vi "GrabNsvReadings.vi"(11 "Simulated Telemetry in":T1 {"Brake Pressure (PSI)" scale=0.0..1000.0; "Maglock 4 (mm)" scale=0.0..15.0; "Maglock 3 (mm)" scale=0.0..15.0; "Maglock 2 (mm)" scale=0.0..15.0; "Maglock 1 (mm)" scale=0.0..15.0; "ToF 4 (mm)" scale=0.0..100.0; "ToF 3 (mm)" scale=0.0..100.0; "ToF 2 (mm)" scale=0.0..100.0; "ToF 1 (mm)" scale=0.0..100.0; "Levitation Pressure (PSI)" scale=0.0..1000.0; "Utility Pressure (PSI)" scale=0.0..1000.0; "Tank Pressure (PSI)" scale=0.0..1000.0; "Brake Voltage (V)" scale=0.0..15.0; "Battery Voltage (V)" scale=0.0..15.0; "Brake Current (A)" scale=0.0..500.0; "Battery Current (A)" scale=0.0..500.0}) -> (3 "Simulated Telemetry out":T1 {"Brake Pressure (PSI)" scale=0.0..1000.0; "Maglock 4 (mm)" scale=0.0..15.0; "Maglock 3 (mm)" scale=0.0..15.0; "Maglock 2 (mm)" scale=0.0..15.0; "Maglock 1 (mm)" scale=0.0..15.0; "ToF 4 (mm)" scale=0.0..100.0; "ToF 3 (mm)" scale=0.0..100.0; "ToF 2 (mm)" scale=0.0..100.0; "ToF 1 (mm)" scale=0.0..100.0; "Levitation Pressure (PSI)" scale=0.0..1000.0; "Utility Pressure (PSI)" scale=0.0..1000.0; "Tank Pressure (PSI)" scale=0.0..1000.0; "Brake Voltage (V)" scale=0.0..15.0; "Battery Voltage (V)" scale=0.0..15.0; "Brake Current (A)" scale=0.0..500.0; "Battery Current (A)" scale=0.0..500.0})   [LabVIEW 2017]
uses:
  Type Defs/prettyTelemetry.ctl
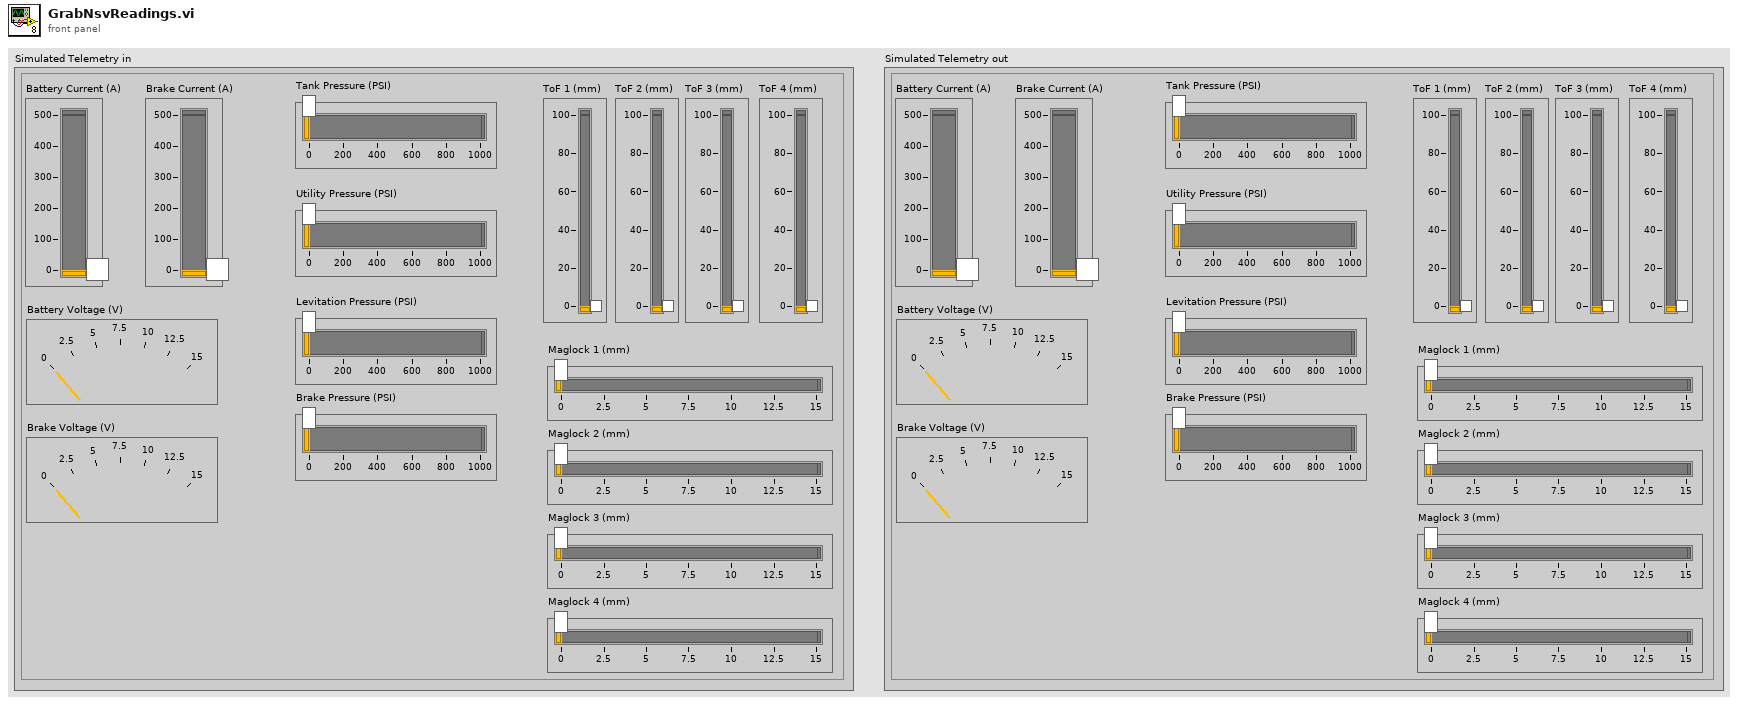
[diagram p1: front panel]
types:
  T1 = typedef "prettyTelemetry.ctl" = cluster{"Battery Current (A)":dbl, "Brake Current (A)":dbl, "Battery Voltage (V)":dbl, "Brake Voltage (V)":dbl, "Tank Pressure (PSI)":dbl, "Utility Pressure (PSI)":dbl, "Levitation Pressure (PSI)":dbl, "Brake Pressure (PSI)":dbl, "ToF 1 (mm)":dbl, "ToF 2 (mm)":dbl, "ToF 3 (mm)":dbl, "ToF 4 (mm)":dbl, "Maglock 1 (mm)":dbl, "Maglock 2 (mm)":dbl, "Maglock 3 (mm)":dbl, "Maglock 4 (mm)":dbl}
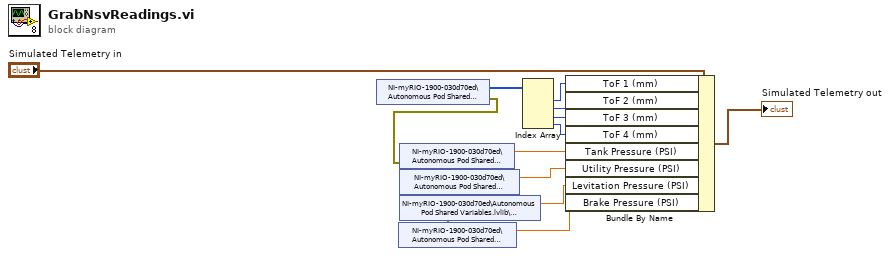
[diagram p0: block diagram]
diagram:
  n1 = shared-variable "NI-myRIO-1900-030d70ed\\Autonomous Pod Shared Variables.lvlib\\ToFReadings"() -> (w9:u8[], error out=w8:errorcluster)  [unwired: 1 in]
  n2 = shared-variable "NI-myRIO-1900-030d70ed\\Autonomous Pod Shared Variables.lvlib\\HighPressure"(error in=w8) -> (w5:dbl, error out=w7:errorcluster)
  n3 = shared-variable "NI-myRIO-1900-030d70ed\\Autonomous Pod Shared Variables.lvlib\\UtilityPressure"(error in=w7) -> (w4:dbl, error out=w6:errorcluster)
  n4 = shared-variable "NI-myRIO-1900-030d70ed\\Autonomous Pod Shared Variables.lvlib\\LevitationPressure"(error in=w6) -> (w3:dbl, error out=w2:errorcluster)
  n5 = shared-variable "NI-myRIO-1900-030d70ed\\Autonomous Pod Shared Variables.lvlib\\BrakePressure"(error in=w2) -> (w1:dbl)  [unwired: 1 out]
  n6 = Index Array(array=w9) -> (element #1=w13:u8, element #2=w12:u8, element #3=w11:u8, element #4=w10:u8)  [unwired: 4 in]
  n7 = Bundle By Name(cluster="Simulated Telemetry in", "ToF 1 (mm)"=w13, "ToF 2 (mm)"=w12, "ToF 3 (mm)"=w11, "ToF 4 (mm)"=w10, "Tank Pressure (PSI)"=w5, "Utility Pressure (PSI)"=w4, "Levitation Pressure (PSI)"=w3, "Brake Pressure (PSI)"=w1) -> (→"Simulated Telemetry out":T1)
